vi "readInEthernetXml.vi"(8 "error in (no error)":errorcluster, 10 "xml in":refnum<class "NativeXML.lvclass">, 11 "deviceDataBase in":refnum<class "deviceDataBase.lvclass">) -> (0 "error out":errorcluster, 1 "device.lvclass out":refnum<class "device.lvclass">, 3 "deviceDataBase out":refnum<class "deviceDataBase.lvclass">)   [LabVIEW 2009, in "Tools.lvlib" / "DatabaseHelpers.lvlib" / "deviceDataBase.lvclass"]
uses:
  deviceDataBase.lvclass
  Database Objects/device/device.lvclass
  NativeXML/NativeXML.lvclass
  Database Objects/device/EthernetSupply/ethernetSupply.lvclass
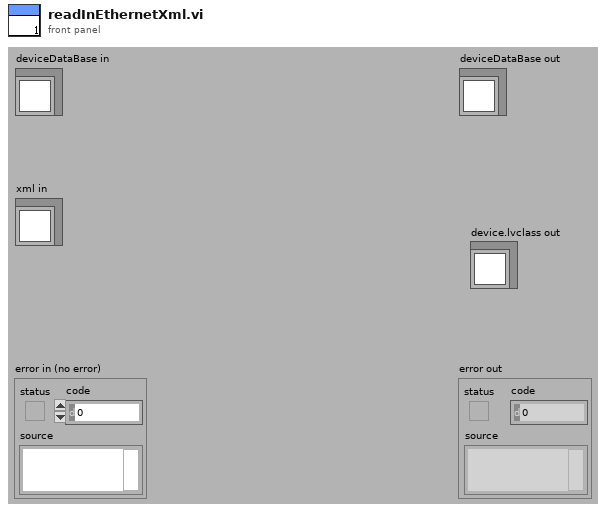
[diagram p1: front panel]
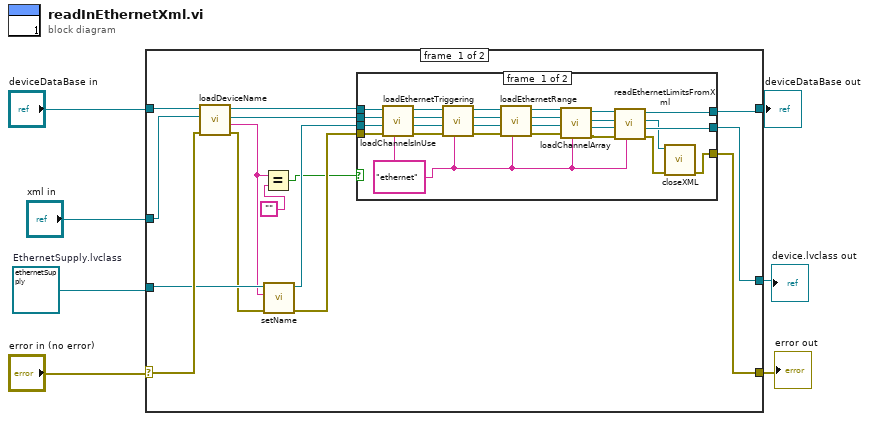
[diagram p0: block diagram]
diagram:
  w1 = refnum<class "ethernetSupply.lvclass"> refnum  # EthernetSupply.lvclass
  n1 = case shown="No Error" "error in (no error)" {
    selector: "error in (no error)" -> [w21 w53]
    tunnel: [w8 w53] -> w5
    tunnel: [w12 w52] -> w4
    tunnel: "deviceDataBase in" -> [w22 w52]
    tunnel: "xml in" -> [w20 _]
    tunnel: w1 -> [w19 _]
    tunnel: [w13 _] -> w3
    frame #0 {
      n2 = call "loadDeviceName.vi"("error in (no error)"=w21, "NativeXML in"=w20, "deviceDataBase in"=w22) -> ("error out"=w18:errorcluster, "deviceName"=w9:string, "NativeXML out"=w15:refnum<class "NativeXML.lvclass">, "deviceDataBase out"=w17:refnum<class "deviceDataBase.lvclass">)  [unwired: 5 in]
      n3 = Equal?(x=w9, y="") -> (x = y?=w11:bool)
      n4 = call "setName.vi"("error in (no error)"=w18, "name"=w9, "device.lvclass in"=w19) -> ("error out"=w16:errorcluster, "device.lvclass out"=w14:refnum<class "ethernetSupply.lvclass">)  [unwired: 7 in]
      n5 = case shown="False" w11 {
        tunnel: w17 -> [w48 w51]
        tunnel: w16 -> [w47 w49]
        tunnel: w15 -> [w46 _]
        tunnel: w14 -> [w45 w50]
        tunnel: [w23 w49] -> w8
        tunnel: [w30 w50] -> w13
        tunnel: [w31 w51] -> w12
        frame #0 {
          w26 = "ethernet"
          n6 = call "loadChannelsInUse.vi"("type"=w26, "error in (no error)"=w47, "device.lvclass"=w45, "NativeXML in"=w46, "deviceDataBase in"=w48) -> ("error out"=w41:errorcluster, "device.lvclass out"=w42:refnum<class "device.lvclass">, "NativeXML out"=w43:refnum<class "NativeXML.lvclass">, "deviceDataBase out"=w44:refnum<class "deviceDataBase.lvclass">)  [unwired: 3 in]
          n7 = call "loadEthernetTriggering.vi"("type"=w26, "error in (no error)"=w41, "device.lvclass"=w42, "xml in"=w43, "deviceDataBase in"=w44) -> ("error out"=w35:errorcluster, "device.lvclass out"=w34:refnum<class "device.lvclass">, "xml out"=w33:refnum<class "NativeXML.lvclass">, "deviceDataBase out"=w40:refnum<class "deviceDataBase.lvclass">)  [unwired: 3 in]
          n8 = call "loadEthernetRange.vi"("type"=w26, "error in (no error)"=w35, "device.lvclass"=w34, "xml in"=w33, "deviceDataBase in"=w40) -> ("error out"=w36:errorcluster, "device.lvclass out"=w37:refnum<class "device.lvclass">, "xml out"=w38:refnum<class "NativeXML.lvclass">, "deviceDataBase out"=w39:refnum<class "deviceDataBase.lvclass">)  [unwired: 3 in]
          n9 = call "loadChannelArray.vi"("type"=w26, "error in (no error)"=w36, "device.lvclass"=w37, "NativeXML in"=w38, "deviceDataBase in"=w39) -> ("error out"=w29:errorcluster, "device.lvclass out"=w28:refnum<class "device.lvclass">, "NativeXML out"=w27:refnum<class "NativeXML.lvclass">, "deviceDataBase out"=w32:refnum<class "deviceDataBase.lvclass">)  [unwired: 3 in]
          n10 = call "readEthernetLimitsFromXml.vi"("type"=w26, "error in (no error)"=w29, "device.lvclass"=w28, "xml in"=w27, "deviceDataBase in"=w32) -> ("error out"=w24:errorcluster, "device.lvclass out"=w30:refnum<class "device.lvclass">, "xml out"=w25:refnum<class "NativeXML.lvclass">, "deviceDataBase out"=w31:refnum<class "deviceDataBase.lvclass">)  [unwired: 3 in]
          n11 = call "closeXML.vi"("error in (no error)"=w24, "NativeXML in"=w25) -> ("error out"=w23:errorcluster)  [unwired: 9 in]
        }
        frame #1 {
        }
      }
    }
    frame #1 {
    }
  }
  "error out" <- w5
  "deviceDataBase out" <- w4
  "device.lvclass out" <- w3
